vi "RedSubVi.vi"(3 "error in (no error)":errorcluster, 4 "Disabled":T1(ring), 5 "Array":refnum<vi>[](array[refnum])) -> (0 "error out":errorcluster, 1 "Output reference":refnum<vi>[](array[refnum]))   [LabVIEW 2017]
doc: "This SubVi will disable all elements recieved in the array input, using a property node"
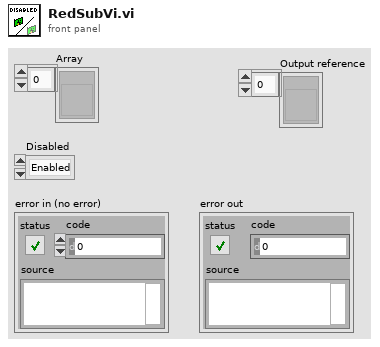
[diagram p1: front panel]
types:
  T1 = enum8{"Enabled", "Disabled", "Disabled and Grayed Out"}
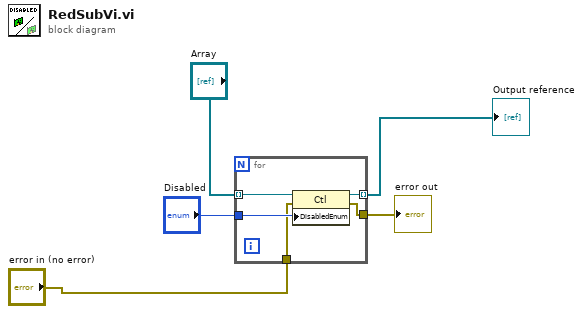
[diagram p0: block diagram]
diagram:
  n1 = for {
    tunnel: "Array" -> [w10] mode=indexing
    tunnel: "Disabled" -> [w9]
    tunnel: "error in (no error)" -> [w8]
    tunnel: [w7] -> w5
    tunnel: [w6] -> w1 mode=indexing
    n2 = property class="Ctl"(reference=w10, error in=w8, "DisabledEnum"=w9) -> (reference out=w6:refnum<vi>, error out=w7:errorcluster)
  }
  "error out" <- w5
  "Output reference" <- w1
